vi "Get Relocated Dependent Modules.vi"(8 "error in (no error)":errorcluster, 11 "Routing and Faulting Ref in":T1 format="%.0x") -> (0 "error out":errorcluster, 1 "Removed Dependent Modules":string[](array[string]), 2 "Outdated Dependent Modules":cluster{"Old Path":string, "New Path":string}[](array[cluster]), 3 "Routing and Faulting Ref out":T1 format="%.0x")   [LabVIEW 2017, in "Routing and Faulting System Explorer.lvlib"]
uses:
  Routing and Faulting System Explorer.lvlib
  <vilib>/NI Veristand/Custom Device API/Custom Device Item Ref.ctl
  Shared/Routing and Faulting Hardware API/Routing and Faulting Hardware API.lvlib
  <vilib>/NI Veristand/Custom Device API/Custom Device API.lvlib
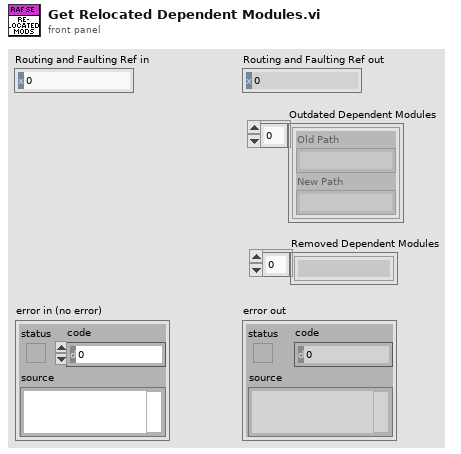
[diagram p1: front panel]
types:
  T1 = typedef "Custom Device API.lvlib/Custom Device Item Ref.ctl" = u64
  T2 = cluster{"Expected Path":string, "Module Ref":T1}[]
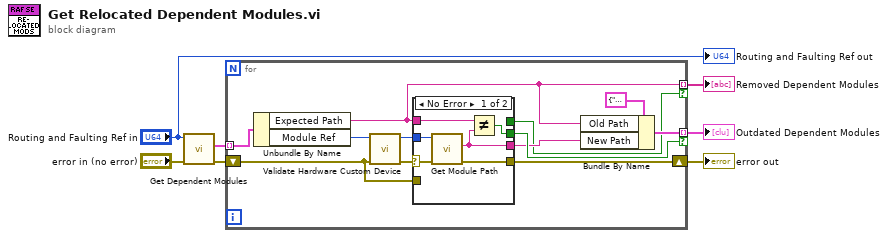
[diagram p0: block diagram]
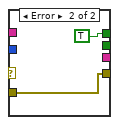
[diagram p2: hidden frame]
diagram:
  n1 = call "Get Dependent Modules.vi"("error in (no error)"="error in (no error)", "Routing and Faulting Ref in"="Routing and Faulting Ref in") -> ("error out"=w4:errorcluster, "Dependent Modules"=w1:T2)  [unwired: 7 in, 1 out]
  n2 = for {
    tunnel: w1 -> [w11] mode=indexing
    shift-right: [w18] -> w7
    shift-left: w4 -> [w8]
    tunnel: [w14] -> w6 mode=indexing if=w16
    tunnel: [w9] -> w5 mode=indexing if=w12
    n3 = Unbundle By Name(w11) -> ("Expected Path"=w9:string, "Module Ref"=w10:T1)
    n4 = call "Validate Hardware Custom Device.vi"("error in (no error)"=w8, "Hardware Ref in"=w10) -> ("error out"=w19:errorcluster, "Hardware Ref out"=w17:T1)  [unwired: 8 in]
    n5 = case shown="No Error" w19 {
      selector: w19 -> [w25 _]
      tunnel: w8 -> [_ w27]
      tunnel: [w21 w27] -> w18
      tunnel: w17 -> [w24 _]
      tunnel: w9 -> [w23 _]
      tunnel: [w22 _] -> w16
      tunnel: [w20 _] -> w13
      tunnel: [_ TRUE] -> w12
      frame No Error {
        n6 = call "Get Module Path.vi"("error in (no error)"=w25, "Hardware Ref in"=w24) -> ("error out"=w21:errorcluster, "Resource"=w20:string)  [unwired: 6 in, 2 out]
        n7 = Not Equal?(x=w23, y=w20) -> (x != y?=w22:bool)
      }
      frame Error {
      }
    }
    n8 = Bundle By Name(cluster=cluster{"Old Path":string, "New Path":string} {"Old Path"="", "New Path"=""} ("input cluster"), "Old Path"=w9, "New Path"=w13) -> (w14:cluster{"Old Path":string, "New Path":string})
  }
  "error out" <- w7
  "Outdated Dependent Modules" <- w6
  "Removed Dependent Modules" <- w5
  "Routing and Faulting Ref out" <- "Routing and Faulting Ref in"
